vi "_PC_Pub_MS_EMA_Process.vi"(7 "Init? ( F )":bool, 8 "error in (no error)":errorcluster, 10 "SigInfo in":T1, 11 "AVGValue":u8) -> (0 "error out":errorcluster, 2 "SigInfo out":T1, 4 "AVG Items":u8)   [LabVIEW 2018]
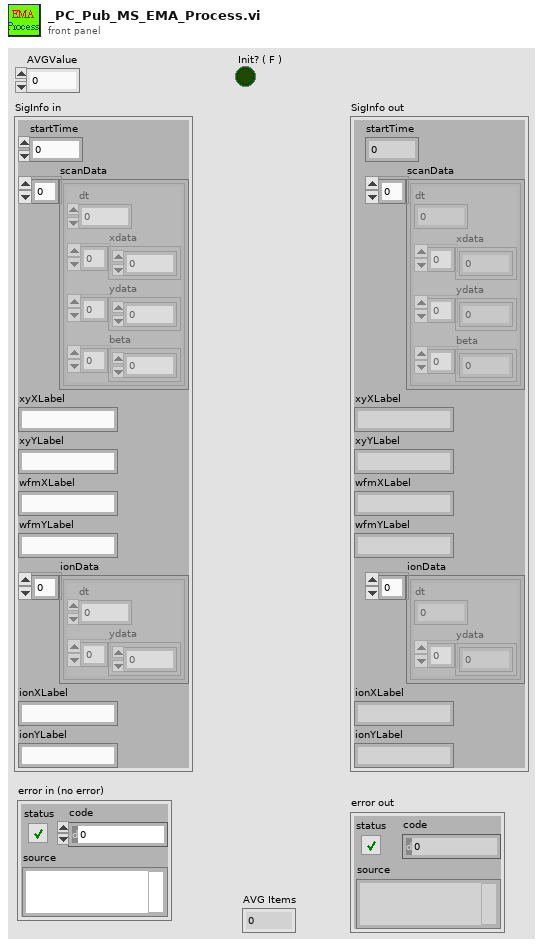
[diagram p1: front panel]
types:
  T1 = cluster{"startTime":dbl, "scanData":cluster{"dt":dbl, "xdata":dbl[], "ydata":sgl[], "beta":dbl[]}[], "xyXLabel":string, "xyYLabel":string, "wfmXLabel":string, "wfmYLabel":string, "ionData":cluster{"dt":dbl, "ydata":sgl[]}[], "ionXLabel":string, "ionYLabel":string}
  T2 = cluster{"EMAPrev out":sgl[], "EMACurrent out":sgl[]}[]
  T3 = cluster{"dt":dbl, "xdata":dbl[], "ydata":sgl[], "beta":dbl[]}[]
  T4 = cluster{"EMAPrev out":sgl[], "EMACurrent out":sgl[]}
  T5 = cluster{"dt":dbl, "xdata":dbl[], "ydata":sgl[], "beta":dbl[]}
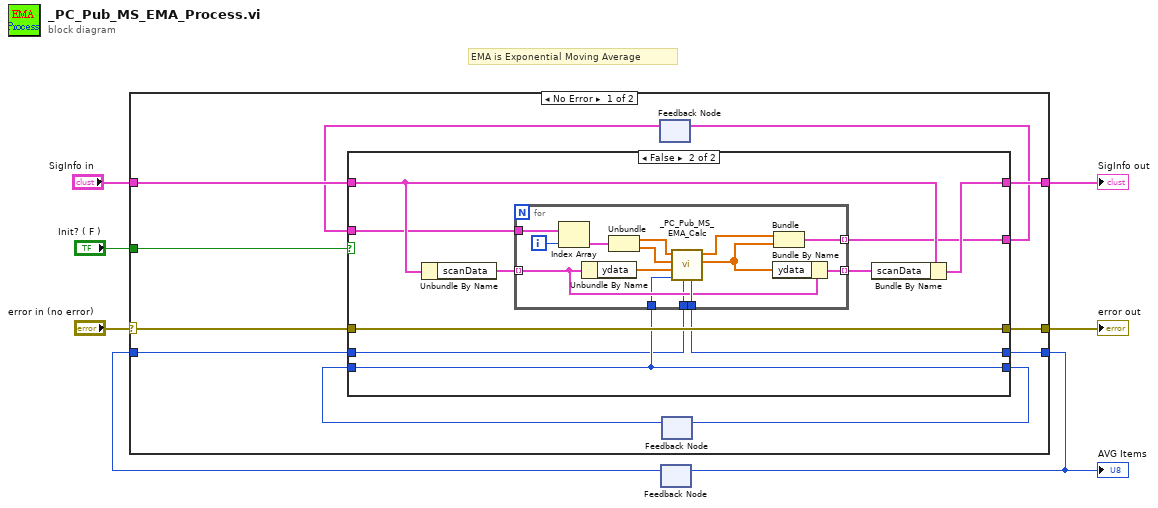
[diagram p0: block diagram]
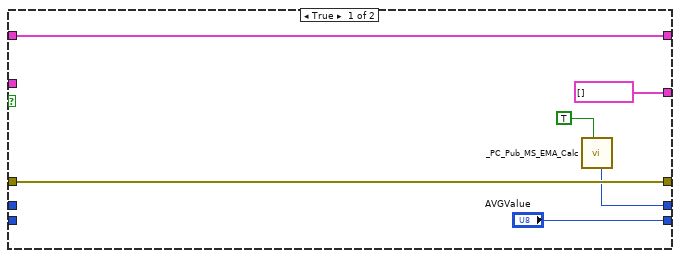
[diagram p2: hidden frame]
diagram:
  # "EMA is Exponential Moving Average"
  n1 = feedback #1() -> (w2:u8)  [unwired: 1 in]
  n2 = case shown="No Error" "error in (no error)" {
    selector: "error in (no error)" -> [w16 w50]
    tunnel: "Init? ( F )" -> [w8 _]
    tunnel: "SigInfo in" -> [w18 w51]
    tunnel: [w17 w51] -> w3
    tunnel: [w15 w50] -> w6
    tunnel: [w13 w49] -> w1
    tunnel: w2 -> [w12 w49]
    frame No Error {
      n3 = feedback #2() -> (w9:T2)  [unwired: 1 in]
      n4 = feedback #3() -> (w11:u8)  [unwired: 1 in]
      n5 = case shown="False" w8 {
        tunnel: [w23 w29] -> w17
        tunnel: w18 -> [w23 w31]
        tunnel: w16 -> [w22 w34]
        tunnel: [w22 w34] -> w15
        tunnel: ["AVGValue" w28] -> w14
        tunnel: w11 -> [_ w28]
        tunnel: [w20 w33] -> w13
        tunnel: w12 -> [_ w27]
        tunnel: [T2 [] w26] -> w10
        tunnel: w9 -> [_ w25]
        frame True {
          n6 = call "_PC_Pub_MS_EMA_Calc.vi"("Init"=TRUE) -> ("AVG Items out"=w20:u8)  [unwired: 8 in, 2 out]
        }
        frame False {
          n7 = Unbundle By Name(w31) -> ("scanData"=w32:T3)
          n8 = for {
            tunnel: w28 -> [w43]
            tunnel: [w48] -> w33
            tunnel: w32 -> [w47] mode=indexing
            tunnel: [w46] -> w30 mode=indexing
            tunnel: w27 -> [w45]
            tunnel: [w41] -> w26 mode=indexing
            tunnel: w25 -> [w38]
            i -> [w39]
            n9 = Index Array(array=w38, index=w39) -> (element=w37:T4)
            n10 = Unbundle By Name(w47) -> ("ydata"=w42:sgl[])
            n11 = Unbundle(w37) -> ("EMAPrev out"=w36:sgl[], "EMACurrent out"=w35:sgl[])
            n12 = call "_PC_Pub_MS_EMA_Calc.vi"("AVG Items in"=w45, "maxItems"=w43, "Y Data"=w42, "EMACurrent in"=w35, "EMAPrev in"=w36) -> ("EMACurrent out"=w40:sgl[], "EMAPrev out"=w44:sgl[], "AVG Items out"=w48:u8)  [unwired: 4 in]
            n13 = Bundle By Name(cluster=w47, "ydata"=w40) -> (w46:T5)
            n14 = Bundle("EMAPrev out"=w44, "EMACurrent out"=w40) -> (w41:T4)  [unwired: 1 in]
          }
          n15 = Bundle By Name(cluster=w31, "scanData"=w30) -> (w29:T1)
        }
      }
      n16 = feedback-in #2(w10) -> ()
      n17 = feedback-in #3(w14) -> ()
    }
    frame Error {
    }
  }
  "error out" <- w6
  "AVG Items" <- w1
  "SigInfo out" <- w3
  n18 = feedback-in #1(w1) -> ()
